vi "KickOutLmtRd.vi"(7 "Update":bool) -> (3 "Pressed?":bool)   [LabVIEW 2015]
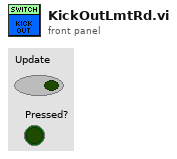
[diagram p1: front panel]
types:
  T1 = typedef "WPI_SwitchDevRef.ctl" = cluster{"DevStatus":errorcluster, "DIO Channel":T2, "CntIndex":T3, "Normally Closed":bool}
  T2 = typedef "FPGA_DIOChannel.ctl" = enum8{"DIO 0", "DIO 1", "DIO 2", "DIO 3", "DIO 4", "DIO 5", "DIO 6", "DIO 7", "DIO 8", "DIO 9", "DIO MXP 0", "DIO MXP 1", "DIO MXP 2", "DIO MXP 3", "DIO MXP 4", "DIO MXP 5", "DIO MXP 6", "DIO MXP 7", "DIO MXP 8", "DIO MXP 9", "DIO MXP 10", "DIO MXP 11", "DIO MXP 12", "DIO MXP 13", "DIO MXP 14", "DIO MXP 15", "Invalid"}
  T3 = typedef "FPGA_CounterCtrSystemIndex.ctl" = enum8{"Ctr 0", "Ctr 1", "Ctr 2", "Ctr 3", "Ctr 4", "Ctr 5", "Ctr 6", "Ctr 7", "Invalid"}
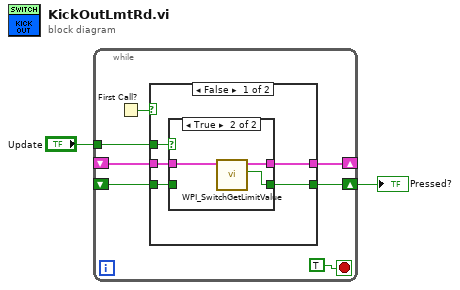
[diagram p0: block diagram]
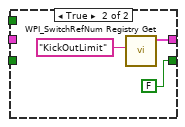
[diagram p3: hidden frame]
diagram:
  n1 = while {
    tunnel: "Update" -> [w7]
    shift-right: [w6] -> _
    shift-left: _ -> [w5]
    shift-right: [w4] -> w1
    shift-left: _ -> [w3]
    stop <- TRUE stop-if-true
    n2 = First Call?() -> (First Call?: T/F=w8:bool)
    n3 = case shown="False" w8 {
      tunnel: w7 -> [w14 _]
      tunnel: [w13 w21] -> w6
      tunnel: w5 -> [w12 _]
      tunnel: [w11 FALSE ("Value")] -> w4
      tunnel: w3 -> [w10 _]
      frame False {
        n4 = case shown="True" w14 {
          tunnel: [w16 w19] -> w13
          tunnel: w12 -> [w16 w18]
          tunnel: [w15 w17] -> w11
          tunnel: w10 -> [w15 _]
          frame False {
          }
          frame True {
            n5 = call <vilib>:"WPI_SwitchGetLimitValue.vi"("SwitchDevRef"=w18) -> ("Switch Pressed"=w17:bool, "SwitchDevRef"=w19:T1)  [unwired: 8 in, 1 out]
          }
        }
      }
      frame True {
        n6 = call <vilib>:"WPI_SwitchRefNum Registry Get.vi"("refnum name"="KickOutLimit") -> ("SwitchDevRef"=w21:T1)  [unwired: 9 in, 1 out]
      }
    }
  }
  "Pressed?" <- w1
